vi "Graph TestRun.vi"(8 "Fehler (Eingang, kein Fehler)":errorcluster) -> (0 "Fehler (Ausgang)":errorcluster, 1 "Max. Wert":i32, 2 "Graph":waveform(dbl)[](array[waveform]), 3 "Messwerte":dbl[](array[numeric]), 5 "Istwerte Kompontente":string[](array[string]))   [LabVIEW 2020, in "EPA 1065.lvlib" / "HovaCAL Interference verificaton.lvlib"]
uses:
  HovaCAL Interference verificaton.lvlib
  Messdaten/Aktionen FGV Messdaten.ctl
  Aktion Index uebersetzten.ctl
  Linearisierung V2/Aktion Lin Daten aufarbeiten.ctl
  Seiten/FT-IR/FGV FT-IR Parameter.vi
  Messdaten/Messdaten.lvlib
  Linearisierung V2/Linearisierung v2.lvlib
  Allgemein/allgemeine Sub-VIs.lvlib
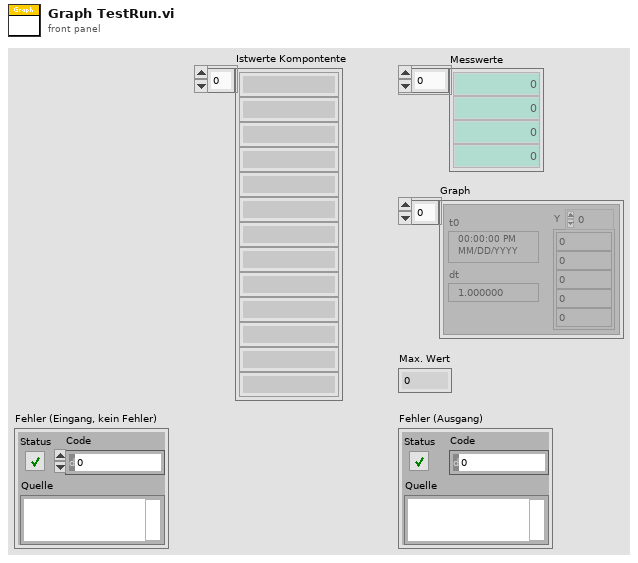
[diagram p1: front panel]
types:
  T1 = typedef "EPA 1065.lvlib/HovaCAL Interference verificaton.lvlib/Aktion Index uebersetzten.ctl" = enum16{"lesen", "schreiben", "auswerten", "Referenzwert", "KompIndex", "RefInterferIndex", "KontrInterfIndex"}
  T2 = typedef "Messdaten.lvlib/Aktionen FGV Messdaten.ctl" = enum16{"lesen", "schreiben", "löschen", "Mittelwerte", "Komponente"}
  T3 = typedef "Linearisierung v2.lvlib/Aktion Lin Daten aufarbeiten.ctl" = enum16{"lesen", "Protkolldaten", "speichern", "laden", "EPA auswerten", "Tabelle schreiben", "Lin auswerten", "Tab init", "Stufentabelle", "EPA aktiviert", "Nachbehandlung laden", "Tabelle löschen", "Istwerte löschen", "Zeile löschen", "Zeile einfügen", "LIN aktiviert", "LIN/EPA aktiv laden", "EGAK Tab", "LIN übernehmen", "Tab init ohne Stufen"}
  T4 = typedef "Linearisierung v2.lvlib/Eingabetabelle.ctl" = string[][]
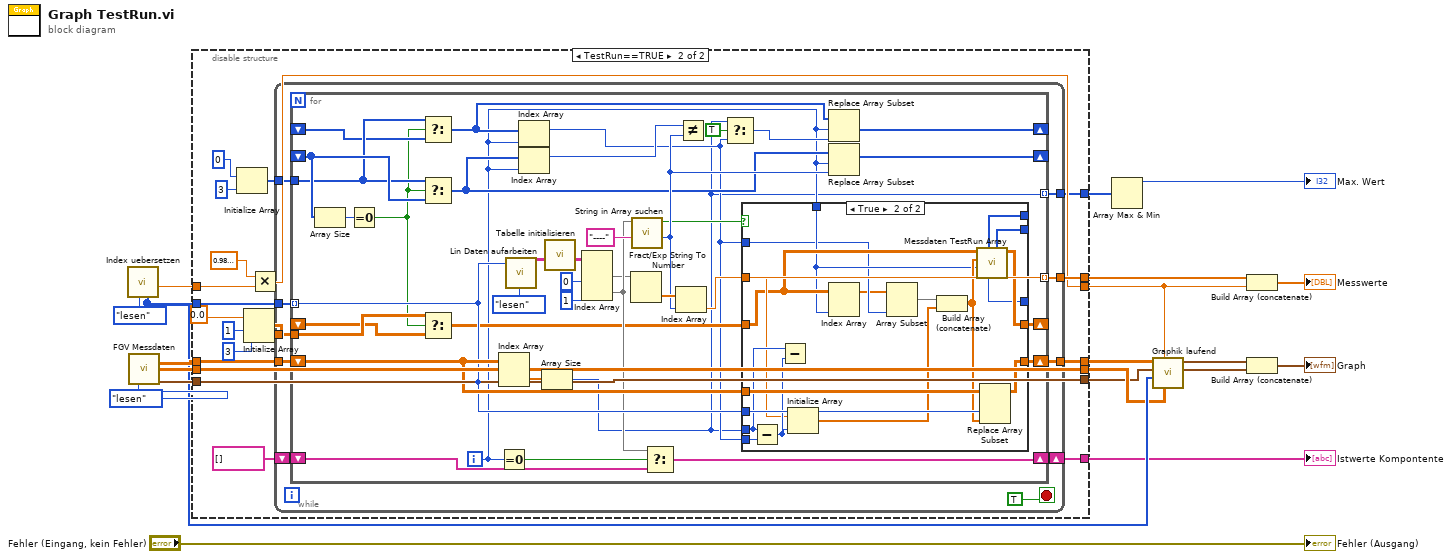
[diagram p0: block diagram]
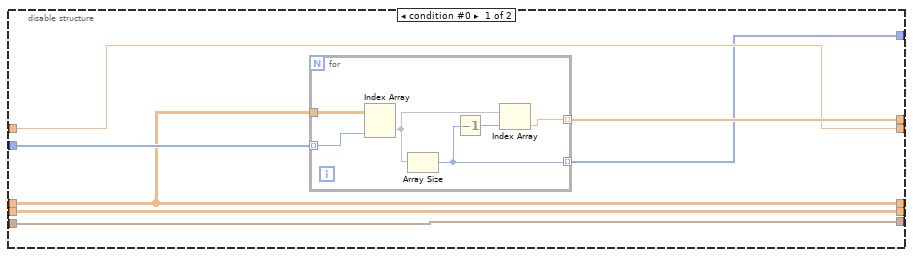
[diagram p2: hidden frame]
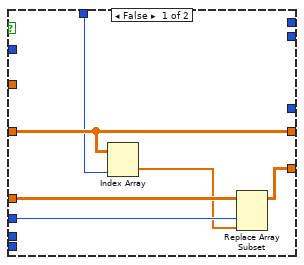
[diagram p3: hidden frame]
diagram:
  n1 = call "Index uebersetzen.vi"("Aktion"=Aktion_Index_uebersetzten."lesen") -> ("Referenz out"=w7:sgl, "Komponenten Indices"=w12:i32[])  [unwired: 5 in, 4 out]
  n2 = call "FGV Messdaten.vi"("Aktionen"=Aktionen_FGV_Messdaten."lesen") -> ("Messdaten"=w19:sgl[][], "Mittelwertdaten"=w18:sgl[][], "Zeitstempeln"=w17:timestamp[])  [unwired: 6 in, 6 out]
  n3 = disable-structure shown="TestRun==TRUE" {
    disable-tunnel: w19 -> [w23 w52]
    disable-tunnel: [w23 w48] -> w2
    disable-tunnel: w18 -> [w27 w50]
    disable-tunnel: [w27 w50] -> w6
    disable-tunnel: w17 -> [w26 w49]
    disable-tunnel: [w26 w49] -> w1
    disable-tunnel: w12 -> [w25 w51]
    disable-tunnel: [w24 w47] -> w9
    disable-tunnel: [_ w45] -> w8
    disable-tunnel: w7 -> [w22 w44]
    disable-tunnel: [w22 w43] -> w3
    disable-tunnel: [w21 w34] -> w5
    frame condition #0 {
      n4 = for {
        tunnel: w25 -> [w32] mode=indexing
        tunnel: [w30] -> w24 mode=indexing
        tunnel: w23 -> [w33]
        tunnel: [w28] -> w21 mode=indexing
        n5 = Index Array(array=w33, index (col)=w32) -> (element=w31:sgl[])  [unwired: 1 in]
        n6 = Array Size(array=w31) -> (size(s)=w28:i32)
        n7 = Decrement(x=w28) -> (x-1=w29:i32)
        n8 = Index Array(array=w31, index=w29) -> (element=w30:sgl)
      }
    }
    frame condition #1 (active) {
      n9 = Initialize Array(0 ("Element"), 3 ("Dimensionsgröße")) -> (w39:i32[])
      n10 = Initialize Array(sgl 0.0 ("Numerisch"), 1 ("Dimensionsgröße"), 3 ("Dimensionsgröße")) -> (w35:sgl[][])
      n11 = Multiply(x=sgl 0.98, y=w44) -> (x*y=w43:sgl)
      n12 = while {
        tunnel: w52 -> [w62]
        tunnel: w51 -> [w61]
        tunnel: [w60] -> w48
        tunnel: [w59] -> w47
        tunnel: w39 -> [w55]
        tunnel: w35 -> [w54]
        shift-right: [w57] -> w45
        shift-left: string[] [] ("Tabelle") -> [w58]
        tunnel: [w53] -> w34
        stop <- TRUE stop-if-true
        n13 = for {
          tunnel: w61 -> [w98] mode=indexing
          shift-right: [w95] -> w60
          shift-left: w62 -> [w100]
          tunnel: [w73] -> w59 mode=indexing
          shift-right: [w92] -> w57
          shift-left: w58 -> [w91]
          shift-right: [w83] -> _
          shift-left: _ -> [w77]
          shift-right: [w84] -> _
          shift-left: _ -> [w74]
          tunnel: w55 -> [w76]
          shift-right: [w71] -> _
          shift-left: _ -> [w68]
          tunnel: w54 -> [w70]
          tunnel: [w63] -> w53 mode=indexing
          i -> [w66]
          n14 = Array Size(array=w77) -> (size(s)=w79:i32)
          n15 = Equal To 0?(x=w79) -> (x = 0?=w69:bool)
          n16 = Select(t=w76, s=w69, f=w74) -> (s? t:f=w75:i32[])
          n17 = Select(t=w76, s=w69, f=w77) -> (s? t:f=w78:i32[])
          n18 = Select(t=w70, s=w69, f=w68) -> (s? t:f=w67:sgl[][])
          n19 = Index Array(array=w100, index (col)=w98) -> (element=w81:sgl[])  [unwired: 1 in]
          n20 = Equal To 0?(x=w66) -> (x = 0?=w93:bool)
          n21 = call "Lin Daten aufarbeiten.vi"("Index (Seite)"=w98, "Aktionen"=Aktion_Lin_Daten_aufarbeiten."lesen") -> ("Eingabetabelle"=w97:T4)  [unwired: 15 in, 10 out]
          n22 = Index Array(array=w75, index=w66) -> (element=w64:i32)
          n23 = Index Array(array=w78, index=w66) -> (element=w85:i32)
          n24 = Array Size(array=w81) -> (size(s)=w63:i32)
          n25 = call "Tabelle initialisieren.vi"("Neue Tabelle"=w97) -> ("Tabelle"=w96:string[][])  [unwired: 10 in]
          n26 = Index Array(array=w96, index (col) #1=0 ("Deaktivierter Index (Spalte)"), index (col) #2=1 ("Index (Spalte)")) -> (element #1=w88:string[], element #2=w89:string[])  [unwired: 2 in]
          n27 = Fract/Exp String To Number(string=w88) -> (number=w94:dbl[])  [unwired: 3 in, 1 out]
          n28 = call "String in Array suchen.vi"("Nach String/Zeichen suchen (-)"="----", "String-Array"=w89) -> ("Index"=w82:i32, "Gefunden?"=w72:bool)  [unwired: 7 in, 1 out]
          n29 = Select(t=w89, s=w93, f=w91) -> (s? t:f=w92:string[])
          n30 = Index Array(array=w94, index=w82) -> (element=w73:dbl)
          n31 = Not Equal?(x=w85, y=w82) -> ()  [unwired: 1 out]
          n32 = Select(t=w63, s=TRUE, f=w64) -> (s? t:f=w80:i32)
          n33 = case shown="True" w72 {
            tunnel: w100 -> [w106 w124]
            tunnel: w98 -> [w104 w123]
            tunnel: [w105 w122] -> w95
            tunnel: w64 -> [_ w121]
            tunnel: w63 -> [_ w120]
            tunnel: w73 -> [_ w118]
            tunnel: [w103 w117] -> w71
            tunnel: w67 -> [w103 w116]
            tunnel: w66 -> [w102 w114]
            tunnel: [_ w113] -> _
            tunnel: [_ w112] -> _
            tunnel: [_ w111] -> _
            tunnel: w64 -> [_ w109]
            frame False {
              n34 = Index Array(array=w103, index (col)=w102) -> (element=w101:sgl[])  [unwired: 1 in]
              n35 = Replace Array Subset(array=w106, new element=w101, index (col)=w104) -> (w105:sgl[][])  [unwired: 1 in]
            }
            frame True {
              n36 = Subtract(x=w120, y=w121) -> (x-y=w119:i32)
              n37 = Subtract(x=w120, y=w119) -> ()  [unwired: 1 out]
              n38 = Initialize Array(w118, w119) -> (w107:dbl[])
              n39 = Index Array(array=w116, index (col)=w114) -> (element=w108:sgl[])  [unwired: 1 in]
              n40 = Array Subset(array=w108, length=w109) -> (w110:sgl[])  [unwired: 1 in]
              n41 = Build Array (concatenate)(w110, w107) -> (w115:dbl[])
              n42 = call "Messdaten TestRun Array.vi"("Index"=w114, "Array (Eingang)"=w115, "Array gesamt (Eingang)"=w116) -> ("Array gesamt (Ausgang)"=w117:sgl[][], "Größe(n) Ausgang"=w112:i32[], "Größe Array"=w111:i32, "Größe(n) Eingang"=w113:i32[])  [unwired: 4 in, 1 out]
              n43 = Replace Array Subset(array=w124, new element=w115, index (col)=w123) -> (w122:sgl[][])  [unwired: 1 in]
            }
          }
          n44 = Replace Array Subset(array=w75, new element=w80, index=w66) -> (w84:i32[])
          n45 = Replace Array Subset(array=w78, new element=w82, index=w66) -> (w83:i32[])
        }
      }
    }
  }
  "Istwerte Kompontente" <- w8
  n46 = Array Max & Min(array=w5) -> (max value=→"Max. Wert":i32)  [unwired: 3 out]
  n47 = call "Graphik laufend.vi"("Mittelwertdaten"=w6, "Numerisch"=w3, "Komponenten Indices"=w12, "Zeitstempeln"=w1, "Messdaten"=w2) -> ("Refernz"=w11:waveform(sgl), "Array"=w15:waveform(dbl)[])  [unwired: 5 in]
  n48 = Build Array (concatenate)(w9, w3) -> (→"Messwerte":dbl[])
  n49 = Build Array (concatenate)(w15, w11) -> (→"Graph":waveform(dbl)[])
  "Fehler (Ausgang)" <- "Fehler (Eingang, kein Fehler)"
